vi "Measurement Logic.vi"(8 "error in":errorcluster, 9 "measurement configuration":T2={"Config Number"=1.2, "Config String"="Lorem ipsum dolor sit"}, 10 "measure call context in":refnum<class "Measure Call Context.lvclass">, 11 "Stop OOB Server UE":refnum<user-event>) -> (0 "error out":errorcluster, 1 "measurement results":T1={"Config Number (Loopback)"=0.0, "Config String (Loopback)"="Empty", "Measurement Logic Counter"=0, "OOB gRPC Port"=0, "PauseResume (Loopback)"=FALSE, "Double (Loopback)"=0.0, "String (Loopback)"="", "Export (Loopback)"=""}, 2 "measure call context out":refnum<class "Measure Call Context.lvclass">)   [LabVIEW 2025, in "Example Plugin.lvclass"]
doc: "Contains the core logic for executing the measurement."
uses:
  Example Plugin.lvclass
  <vilib>/Plug-In SDKs/Measurements/Measure Call Context/Measure Call Context.lvclass
  Measurement Configuration.ctl
  Measurement Results.ctl
  Example Plugin.lvclass/Example Plugin.ctl
  OOB Data Transfer/OOB Data Transfer.lvlib
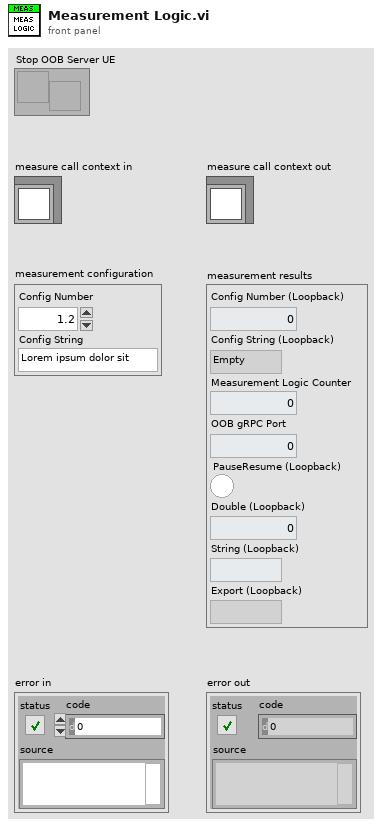
[diagram p1: front panel]
types:
  T1 = typedef "Example Plugin.lvclass/Measurement Results.ctl" = cluster{"Config Number (Loopback)":dbl, "Config String (Loopback)":string, "Measurement Logic Counter":i32, "OOB gRPC Port":i32, "PauseResume (Loopback)":bool, "Double (Loopback)":dbl, "String (Loopback)":string, "Export (Loopback)":string}
  T2 = typedef "Example Plugin.lvclass/Measurement Configuration.ctl" = cluster{"Config Number":dbl, "Config String":string}
  T3 = typedef "OOB Data Transfer.lvlib/OOB to Logic Data.ctl" = cluster{"PauseResume":bool, "Export":string, "Double":dbl, "String":string}
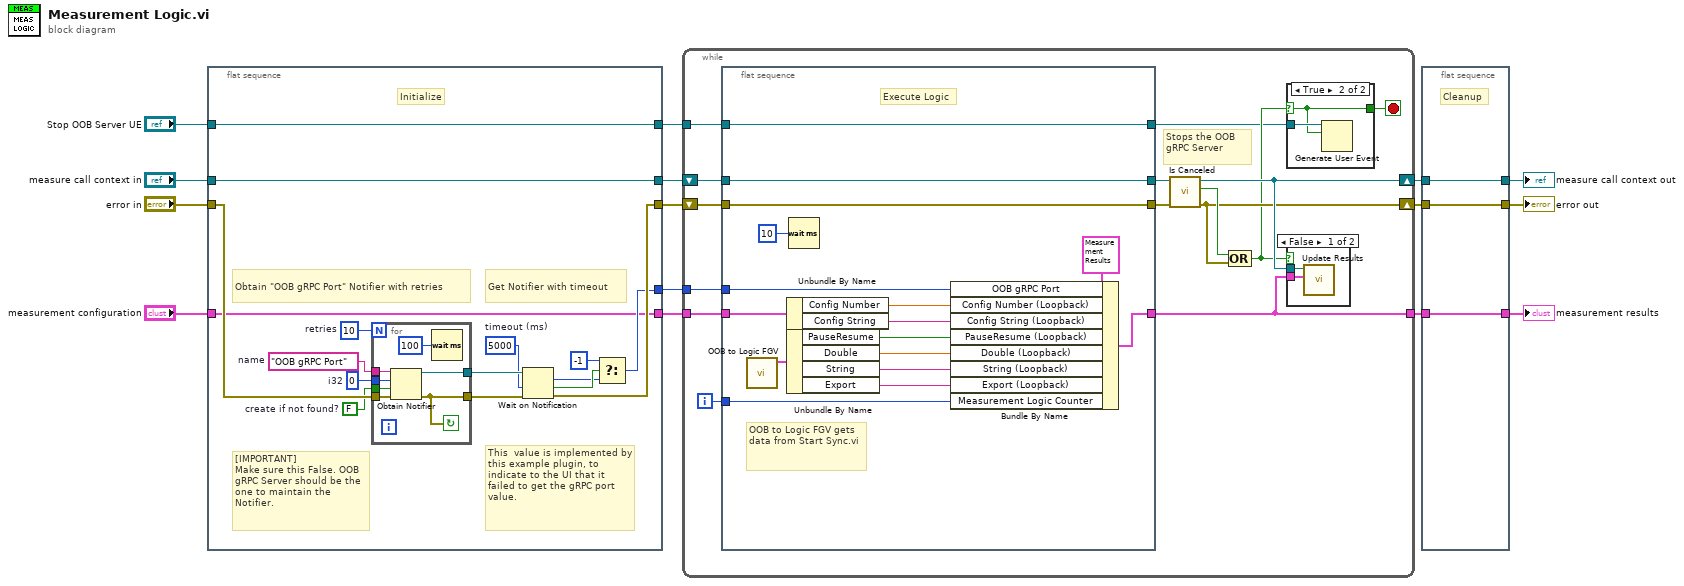
[diagram p0: block diagram]
diagram:
  n1 = flat-sequence {
    tunnel: "error in" -> [w26]
    tunnel: [w24] -> w14
    tunnel: [w23] -> w13
    tunnel: "measurement configuration" -> [w19]
    tunnel: [w19] -> w11
    tunnel: "Stop OOB Server UE" -> [w18]
    tunnel: [w18] -> w9
    tunnel: "measure call context in" -> [w17]
    tunnel: [w17] -> w7
    frame #0 {
      w16 = FALSE  # create if not found?
      w27 = 0  # i32
      w25 = "OOB gRPC Port"  # name
      w28 = 10  # retries
      w29 = 5000  # timeout (ms)
      # "This  value is implemented by this example plugin, to indicate to the UI that it failed to get the gRPC port value."
      # "[IMPORTANT] \nMake sure this False. OOB gRPC Server should be the one to maintain the Notifier."
      # "Initialize"
      # "Obtain \"OOB gRPC Port\" Notifier with retries"
      # "Get Notifier with timeout"
      n2 = for {
        N: w28 -> [_]
        tunnel: [w36] -> w31
        tunnel: [w38] -> w30
        tunnel: w25 -> [w35]
        tunnel: w27 -> [w34]
        tunnel: w26 -> [w33]
        tunnel: w16 -> [w32]
        stop <- w36 continue-if-true
        n3 = Obtain Notifier(name (unnamed)=w35, notification data type=w34, create if not found? (T)=w32, error in (no error)=w33) -> (notifier out=w38:refnum<notifier>, error out=w36:errorcluster)  [unwired: 1 out]
        n4 = Wait (ms)(milliseconds to wait=u32 100) -> ()  [unwired: 1 out]
      }
      n5 = Wait on Notification(notifier=w30, timeout in ms (-1)=w29, error in (no error)=w31) -> (notification=w21:i32, timed out?=w22:bool, error out=w24:errorcluster)  [unwired: 1 in, 1 out]
      n6 = Select(t=-1, s=w22, f=w21) -> (s? t:f=w23:i32)
    }
  }
  n7 = while {
    tunnel: w11 -> [w53]
    tunnel: [w51] -> w5
    shift-right: [w49] -> w6
    shift-left: w7 -> [w40]
    shift-right: [w47] -> w4
    shift-left: w14 -> [w52]
    tunnel: w9 -> [w42]
    tunnel: w13 -> [w44]
    i -> [w43]
    stop <- w45 stop-if-true
    # "Stops the OOB gRPC Server"
    n8 = flat-sequence {
      tunnel: w53 -> [w68]
      tunnel: [w71] -> w51
      tunnel: w52 -> [w74]
      tunnel: [w74] -> w50
      tunnel: w44 -> [w65]
      tunnel: w43 -> [w64]
      tunnel: w42 -> [w60]
      tunnel: [w60] -> w41
      tunnel: w40 -> [w59]
      tunnel: [w59] -> w39
      frame #0 {
        # "OOB to Logic FGV gets data from Start Sync.vi"
        # "Execute Logic"
        n9 = call "OOB to Logic FGV.vi"() -> ("OOB to Logic Data out"=w73:T3)  [unwired: 10 in, 1 out]
        n10 = Unbundle By Name(w68) -> ("Config Number"=w70:dbl, "Config String"=w69:string)
        n11 = Unbundle By Name(w73) -> ("PauseResume"=w67:bool, "Double"=w63:dbl, "String"=w62:string, "Export"=w66:string)
        n12 = Wait (ms)(milliseconds to wait=u32 10) -> ()  [unwired: 1 out]
        n13 = Bundle By Name(cluster=T1 {"Config Number (Loopback)"=0.0, "Config String (Loopback)"="Empty", "Measurement Logic Counter"=0, "OOB gRPC Port"=0, "PauseResume (Loopback)"=FALSE, "Double (Loopback)"=0.0, "String (Loopback)"="", "Export (Loopback)"=""} ("Measurement Results"), "OOB gRPC Port"=w65, "Config Number (Loopback)"=w70, "Config String (Loopback)"=w69, "PauseResume (Loopback)"=w67, "Double (Loopback)"=w63, "String (Loopback)"=w62, "Export (Loopback)"=w66, "Measurement Logic Counter"=w64) -> (w71:T1)
      }
    }
    n14 = call <vilib>:"Is Canceled.vi"("error in"=w50, "measure call context in"=w39) -> ("error out"=w47:errorcluster, "is canceled?"=w48:bool, "measure call context out"=w49:refnum<class "Measure Call Context.lvclass">)  [unwired: 7 in]
    n15 = Compound Arithmetic op=OR(w48, w47) -> (w46:bool)
    n16 = case shown="True" w46 {
      selector: w46 -> [w54 w55]
      tunnel: w41 -> [_ w56]
      tunnel: [w54 w55] -> w45
      frame False {
      }
      frame True {
        n17 = Generate User Event(user event=w56, event data cluster=w55) -> ()  [unwired: 2 in, 2 out]
      }
    }
    n18 = case shown="False" w46 {
      tunnel: w49 -> [w58 _]
      tunnel: w51 -> [w57 _]
      frame False {
        n19 = call <vilib>:"Update Results.vi"("measurement results"=w57, "measure call context in"=w58) -> ()  [unwired: 8 in, 2 out]
      }
      frame True {
      }
    }
  }
  n20 = flat-sequence {
    tunnel: w4 -> [w77]
    tunnel: [w77] -> w2
    tunnel: w5 -> [w76]
    tunnel: [w76] -> w1
    tunnel: w6 -> [w75]
    tunnel: [w75] -> w3
    frame #0 {
      # "Cleanup"
    }
  }
  "error out" <- w2
  "measure call context out" <- w3
  "measurement results" <- w1
